vi "SVT Rolling-Element Bearing.vi"(0 "nominal speed [RPM]":dbl=1200.0 min=0.0, 1 "desired units":u16(ring) items=["Hz", "Order"], 5 "bearing parameters":T1={"number of rolling elements"=8, "pitch diameter"=1.0, "ball/roller diameter"=0.2, "contact angle [deg]"=0.0}, 11 "error in (no error)":errorcluster) -> (4 "outer race frequency":dbl=64.0, 6 "inner race frequency":dbl=96.0, 8 "fundamental train frequency":dbl=8.0, 10 "ball spin frequency":dbl=48.0, 15 "error out":errorcluster)   [LabVIEW 2017, in "SoundVib_MachineCharacteristic.lvlib"]
doc: "Calculates characteristic frequencies or orders of rolling-element bearings or hydrodynamic journal bearings. You must manually select the polymorphic instance you want to use."
uses:
  <vilib>/addons/Sound and Vibration/svt_Machine Characteristic/SoundVib_MachineCharacteristic.lvlib
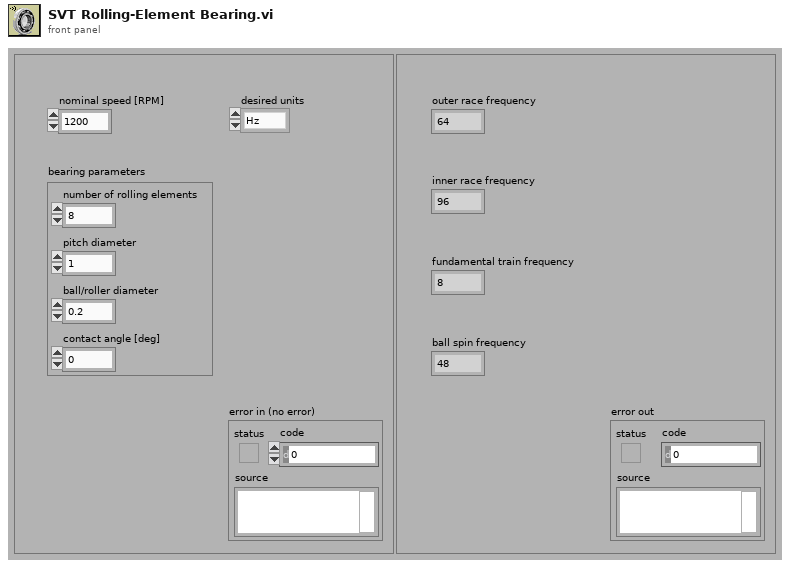
[diagram p1: front panel]
types:
  T1 = cluster{"number of rolling elements":u32, "pitch diameter":dbl, "ball/roller diameter":dbl, "contact angle [deg]":dbl}
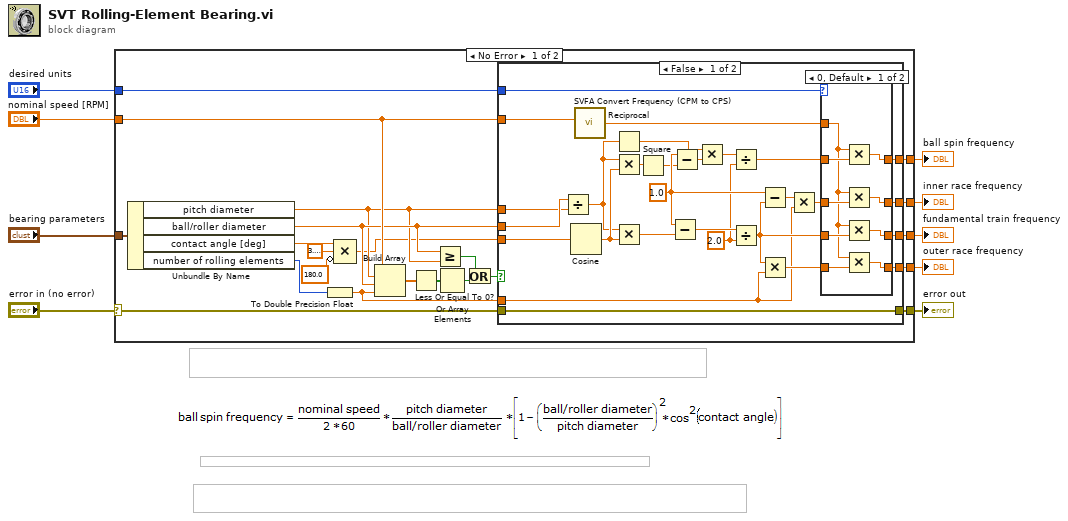
[diagram p0: block diagram]
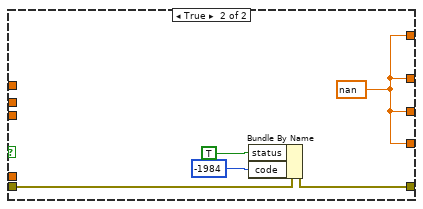
[diagram p3: hidden frame]
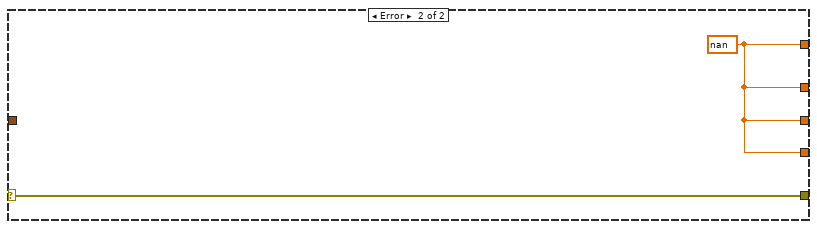
[diagram p4: hidden frame]
diagram:
  n1 = case shown="No Error" "error in (no error)" {
    selector: "error in (no error)" -> [w29 w79]
    tunnel: [w28 w79] -> w8
    tunnel: "bearing parameters" -> [w27 _]
    tunnel: "nominal speed [RPM]" -> [w24 _]
    tunnel: [w26 w78] -> w5
    tunnel: "desired units" -> [w25 _]
    tunnel: [w23 w78] -> w3
    tunnel: [w22 w78] -> w2
    tunnel: [w21 w78] -> w1
    frame No Error {
      n2 = Unbundle By Name(w27) -> ("pitch diameter"=w17:dbl, "ball/roller diameter"=w18:dbl, "contact angle [deg]"=w11:dbl, "number of rolling elements"=w20:u32)
      n3 = To Double Precision Float(number=w20) -> (double precision float=w19:dbl)
      n4 = Compound Arithmetic op=MULTIPLY(w11, 3.141592653589793, invert 180.0 ("value")) -> (w10:dbl)
      n5 = Build Array(w24, w17, w18, w19) -> (w31:dbl[])
      n6 = Less Or Equal To 0?(x=w31) -> (x <= 0?=w30:bool[])
      n7 = Greater Or Equal?(x=w18, y=w17) -> (x >= y?=w15:bool)
      n8 = Or Array Elements(Boolean array=w30) -> (logical OR=w16:bool)
      n9 = Or(x=w15, y=w16) -> (x .or. y?=w14:bool)
      n10 = case shown="False" w14 {
        tunnel: w29 -> [w53 w77]
        tunnel: [w53 w76] -> w28
        tunnel: w18 -> [w59 _]
        tunnel: w17 -> [w58 _]
        tunnel: [w55 w73] -> w26
        tunnel: w25 -> [w54 _]
        tunnel: w24 -> [w41 _]
        tunnel: [w49 w73] -> w23
        tunnel: w19 -> [w44 _]
        tunnel: [w47 w73] -> w22
        tunnel: [w42 w73] -> w21
        tunnel: w10 -> [w32 _]
        frame False {
          w38 = 1.0 ("x")
          w35 = 2.0 ("y")
          n11 = Divide(x=w59, y=w58) -> (x/y=w33:dbl)
          n12 = Cosine(x=w32) -> (cos(x)=w52:dbl)
          n13 = call <vilib>:"SVFA Convert Frequency (CPM to CPS).vi"("nominal speed [RPM]"=w41) -> ("frequency [Hz]"=w40:dbl)  [unwired: 5 in]
          n14 = Reciprocal(x=w33) -> (1/x=w39:dbl)
          n15 = Multiply(x=w33, y=w52) -> (x*y=w37:dbl)
          n16 = Multiply(x=w33, y=w52) -> (x*y=w57:dbl)
          n17 = Square(x=w37) -> (x^2=w36:dbl)
          n18 = Subtract(x=w38, y=w57) -> (x-y=w56:dbl)
          n19 = Subtract(x=w38, y=w36) -> (x-y=w51:dbl)
          n20 = Multiply(x=w39, y=w51) -> (x*y=w34:dbl)
          n21 = Divide(x=w34, y=w35) -> (x/y=w50:dbl)
          n22 = Divide(x=w56, y=w35) -> (x/y=w46:dbl)
          n23 = Subtract(x=w38, y=w46) -> (x-y=w45:dbl)
          n24 = Multiply(x=w46, y=w44) -> (x*y=w48:dbl)
          n25 = Multiply(x=w45, y=w44) -> (x*y=w43:dbl)
          n26 = case shown="0, Default" w54 {
            tunnel: w46 -> [w68 w72]
            tunnel: [w67 w72] -> w55
            tunnel: w40 -> [w60 _]
            tunnel: [w65 w71] -> w49
            tunnel: w50 -> [w66 w71]
            tunnel: w48 -> [w62 w70]
            tunnel: [w61 w70] -> w47
            tunnel: w43 -> [w64 w69]
            tunnel: [w63 w69] -> w42
            frame 0, Default {
              n27 = Multiply(x=w60, y=w66) -> (x*y=w65:dbl)
              n28 = Multiply(x=w60, y=w64) -> (x*y=w63:dbl)
              n29 = Multiply(x=w60, y=w68) -> (x*y=w67:dbl)
              n30 = Multiply(x=w60, y=w62) -> (x*y=w61:dbl)
            }
            frame 1 {
            }
          }
        }
        frame True {
          w73 = nan ("value")
          n31 = Bundle By Name(cluster=w77, "status"=TRUE, "code"=-1984) -> (w76:errorcluster)
        }
      }
    }
    frame Error {
      w78 = nan ("value")
    }
  }
  "outer race frequency" <- w2
  "inner race frequency" <- w1
  "fundamental train frequency" <- w5
  "ball spin frequency" <- w3
  "error out" <- w8
